vi "case 2.vi"() -> ()   [LabVIEW 2016]
panel:
  out "Numeric Indicator":dbl
  in  "b":dbl
  in  "a":dbl
  in  "Enum":T1(ring)
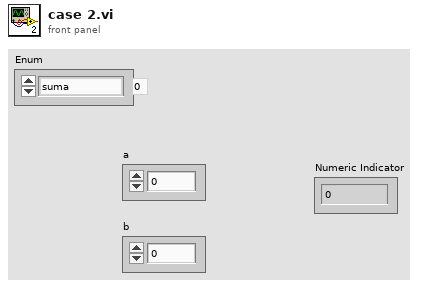
[diagram p1: front panel]
types:
  T1 = enum16{"suma", "resta", "multiplicacion", "divicion"}
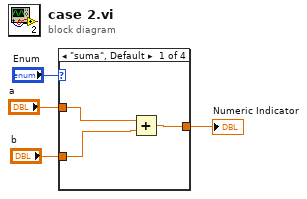
[diagram p0: block diagram]
diagram:
  n1 = case shown="\"suma\", Default" "Enum" {
    tunnel: "a" -> [w7 _ _ _]
    tunnel: "b" -> [w6 _ _ _]
    tunnel: [w5 _ _ _] -> w1
    frame "suma", Default {
      n2 = Add(x=w7, y=w6) -> (x+y=w5:dbl)
    }
    frame "resta" {
    }
    frame "multiplicacion" {
    }
    frame "divicion" {
    }
  }
  "Numeric Indicator" <- w1
